vi "save_config.vi"   [LabVIEW 2011]
doc: "Illustrates how to create and write a configuration settings file.\n\nInstructions:\nEnter values in the controls on the front panel then click on the Run Arrow.\nTo read the file, run Read Configuration Settings File.vi located in the file\\config.llb."
uses:
  global.vi
  <vilib>/Utility/config.llb/Write Key (I32).vi
  <vilib>/Utility/config.llb/Write Key (Boolean).vi
  <vilib>/Utility/config.llb/Write Key (Double).vi
  <vilib>/Utility/config.llb/Write Key (String).vi
  <vilib>/Utility/config.llb/NI_LVConfig.lvlib
types:
  T1 = typedef "NI_LVConfig.lvlib/Config Data RefNum.ctl" = refnum<k1>
  T2 = typedef "scale.ctl" = dbl
  T3 = typedef "sampling_rate.ctl" = ext
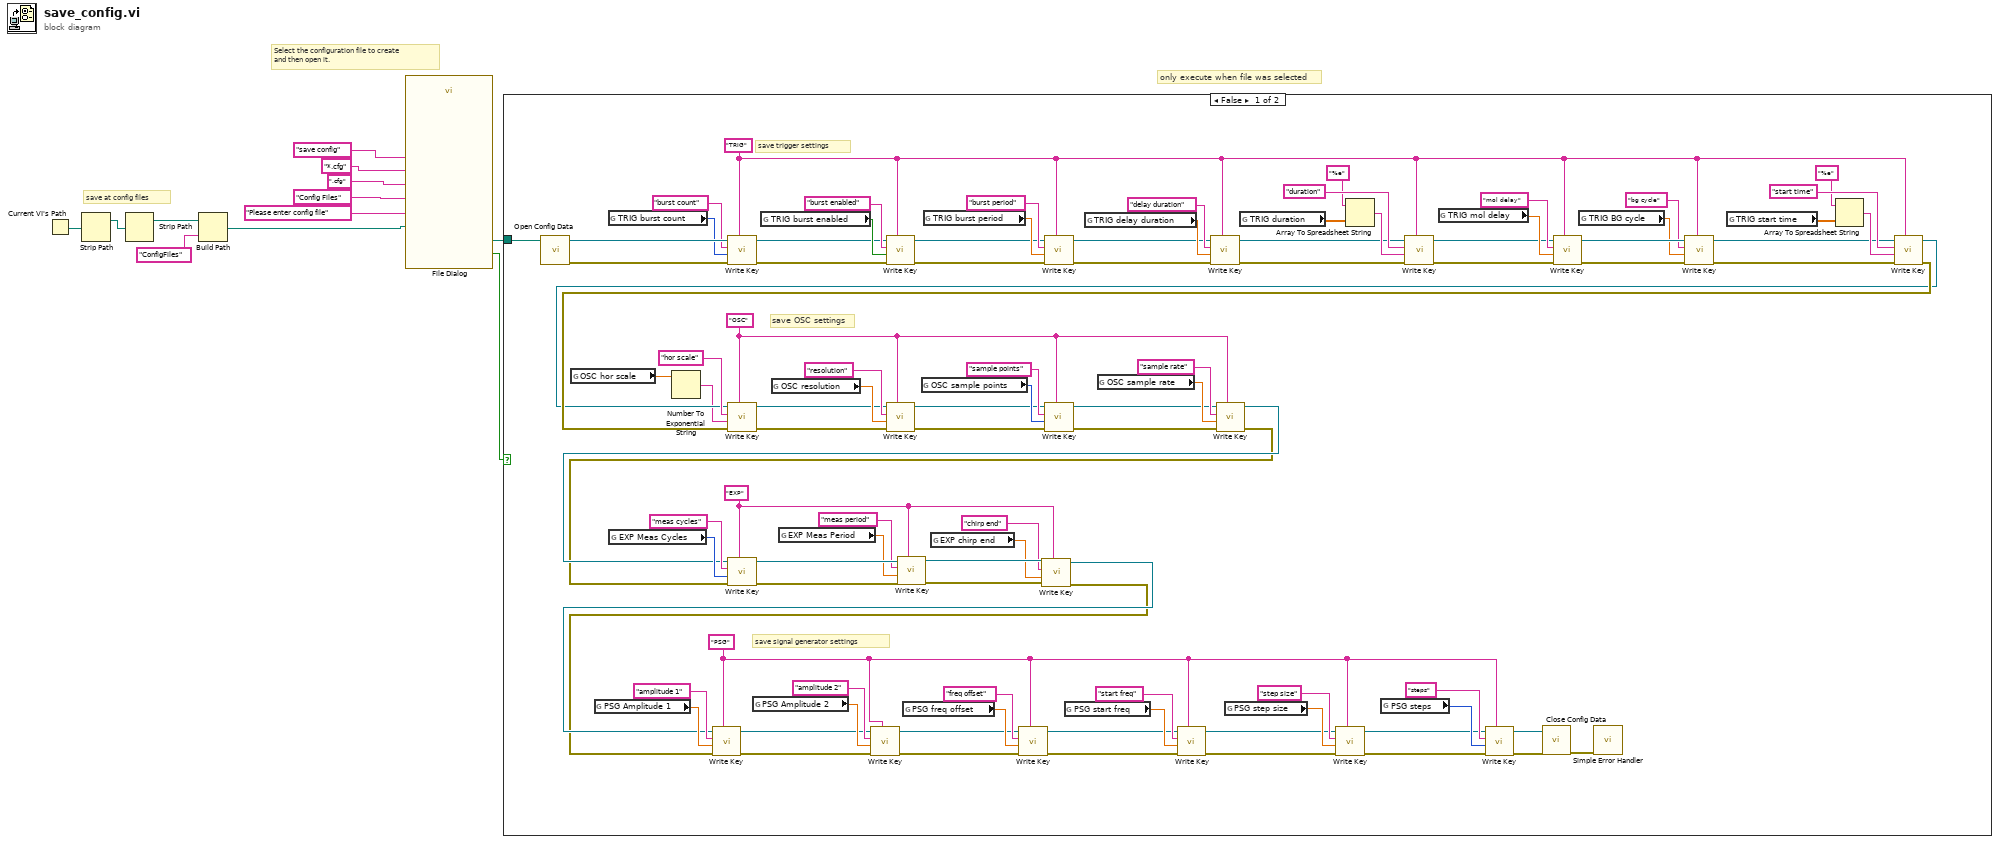
[diagram p0: block diagram]
diagram:
  # "only execute when file was selected"
  # "save at config files"
  # "Select the configuration file to create\nand then open it."
  n1 = Current VI's Path() -> (path=w6:path)
  n2 = Strip Path(path=w6) -> (stripped path=w3:path)  [unwired: 1 out]
  n3 = Strip Path(path=w3) -> (stripped path=w2:path)  [unwired: 1 out]
  n4 = Build Path(base path=w2, name or relative path="ConfigFiles") -> (appended path=w4:path)
  n5 = call "File Dialog"("start path"=w4, "prompt"="Please enter config file", "button label"="save config", "default name"=".cfg", "pattern (all files)"="*.cfg", "pattern label"="Config Files") -> ("selected path"=w12:path, "cancelled"=w1:bool)  [unwired: 6 in, 2 out]
  n6 = case shown="False" w1 {
    tunnel: w12 -> [w105 _]
    frame False {
      w32 = "PSG"
      w15 = "EXP"
      w61 = "OSC"
      w22 = "TRIG"
      # "save signal generator settings"
      # "save OSC settings"
      # "save trigger settings"
      n7 = call <vilib>:"Open Config Data.vi"("configuration file path"=w105) -> ("error out"=w108:errorcluster, "refnum"=w109:T1)  [unwired: 2 in, 7 out]
      n8 = global read "global.vi" "OSC hor scale"() -> (w31:T2)
      n9 = global read "global.vi" "PSG Amplitude 1"() -> (w42:dbl)
      n10 = global read "global.vi" "TRIG burst count"() -> (w104:i32)
      n11 = global read "global.vi" "EXP Meas Cycles"() -> (w59:i32)
      n12 = Number To Exponential String(number=w31) -> (E-format string=w30:string)  [unwired: 3 in]
      n13 = call-poly <vilib>:"Write Key.vi"("section"=w22, "error in (no error)"=w108, "value"=w104, "key"="burst count" ("Key 1"), "refnum"=w109) -> ("error out"=w89:errorcluster, "refnum out"=w93:T1)  [unwired: 5 out]
      n14 = global read "global.vi" "PSG Amplitude 2"() -> (w40:dbl)
      n15 = global read "global.vi" "TRIG burst enabled"() -> (w102:bool)
      n16 = global read "global.vi" "OSC resolution"() -> (w74:ext)
      n17 = global read "global.vi" "EXP Meas Period"() -> (w26:dbl)
      n18 = call-poly <vilib>:"Write Key.vi"("section"=w22, "error in (no error)"=w89, "value"=w102, "key"="burst enabled" ("Key 1"), "refnum"=w93) -> ("error out"=w88:errorcluster, "refnum out"=w92:T1)  [unwired: 5 out]
      n19 = global read "global.vi" "PSG freq offset"() -> (w55:dbl)
      n20 = global read "global.vi" "OSC sample points"() -> (w72:i32)
      n21 = global read "global.vi" "TRIG burst period"() -> (w100:dbl)
      n22 = global read "global.vi" "EXP chirp end"() -> (w13:dbl)
      n23 = call-poly <vilib>:"Write Key.vi"("section"=w22, "error in (no error)"=w88, "value"=w100, "key"="burst period" ("Key 1"), "refnum"=w92) -> ("error out"=w87:errorcluster, "refnum out"=w91:T1)  [unwired: 3 in, 2 out]
      n24 = global read "global.vi" "PSG start freq"() -> (w53:dbl)
      n25 = global read "global.vi" "TRIG delay duration"() -> (w98:dbl)
      n26 = global read "global.vi" "OSC sample rate"() -> (w64:T3)
      n27 = call-poly <vilib>:"Write Key.vi"("section"=w22, "error in (no error)"=w87, "value"=w98, "key"="delay duration" ("Key 1"), "refnum"=w91) -> ("error out"=w86:errorcluster, "refnum out"=w90:T1)  [unwired: 3 in, 2 out]
      n28 = global read "global.vi" "PSG step size"() -> (w51:dbl)
      n29 = global read "global.vi" "TRIG duration"() -> (w95:dbl[])
      n30 = Array To Spreadsheet String(array=w95, 3:"%e" ("format string")) -> (spreadsheet string=w94:string)  [unwired: 1 in]
      n31 = global read "global.vi" "PSG steps"() -> (w45:i32)
      n32 = call-poly <vilib>:"Write Key.vi"("section"=w22, "error in (no error)"=w86, "value"=w94, "key"="duration" ("Key 1"), "refnum"=w90) -> ("error out"=w78:errorcluster, "refnum out"=w79:T1)  [unwired: 1 in, 4 out]
      n33 = global read "global.vi" "TRIG mol delay"() -> (w80:dbl)
      n34 = call-poly <vilib>:"Write Key.vi"("section"=w22, "error in (no error)"=w78, "value"=w80, "key"="mol delay" ("Key 1"), "refnum"=w79) -> ("error out"=w77:errorcluster, "refnum out"=w24:T1)  [unwired: 3 in, 2 out]
      n35 = global read "global.vi" "TRIG BG cycle"() -> (w20:dbl)
      n36 = call-poly <vilib>:"Write Key.vi"("section"=w22, "error in (no error)"=w77, "value"=w20, "key"="bg cycle" ("Key 1"), "refnum"=w24) -> ("error out"=w25:errorcluster, "refnum out"=w23:T1)  [unwired: 4 in, 1 out]
      n37 = global read "global.vi" "TRIG start time"() -> (w83:dbl[])
      n38 = Array To Spreadsheet String(array=w83, 3:"%e" ("format string")) -> (spreadsheet string=w82:string)  [unwired: 1 in]
      n39 = call-poly <vilib>:"Write Key.vi"("section"=w22, "error in (no error)"=w25, "value"=w82, "key"="start time" ("Key 1"), "refnum"=w23) -> ("error out"=w67:errorcluster, "refnum out"=w66:T1)  [unwired: 1 in, 4 out]
      n40 = call-poly <vilib>:"Write Key.vi"("section"=w61, "error in (no error)"=w67, "value"=w30, "key"="hor scale" ("Key 1"), "refnum"=w66) -> ("error out"=w69:errorcluster, "refnum out"=w71:T1)  [unwired: 1 in, 4 out]
      n41 = call-poly <vilib>:"Write Key.vi"("section"=w61, "error in (no error)"=w69, "value"=w74, "key"="resolution" ("Key 1"), "refnum"=w71) -> ("error out"=w68:errorcluster, "refnum out"=w70:T1)  [unwired: 3 in, 2 out]
      n42 = call-poly <vilib>:"Write Key.vi"("section"=w61, "error in (no error)"=w68, "value"=w72, "key"="sample points" ("Key 1"), "refnum"=w70) -> ("error out"=w62:errorcluster, "refnum out"=w63:T1)  [unwired: 5 out]
      n43 = call-poly <vilib>:"Write Key.vi"("section"=w61, "error in (no error)"=w62, "value"=w64, "key"="sample rate" ("Key 1"), "refnum"=w63) -> ("error out"=w57:errorcluster, "refnum out"=w58:T1)  [unwired: 3 in, 2 out]
      n44 = call-poly <vilib>:"Write Key.vi"("section"=w15, "error in (no error)"=w57, "value"=w59, "key"="meas cycles" ("Key 1"), "refnum"=w58) -> ("error out"=w28:errorcluster, "refnum out"=w29:T1)  [unwired: 5 out]
      n45 = call-poly <vilib>:"Write Key.vi"("section"=w15, "error in (no error)"=w28, "value"=w26, "key"="meas period" ("Key 1"), "refnum"=w29) -> ("error out"=w18:errorcluster, "refnum out"=w19:T1)  [unwired: 3 in, 2 out]
      n46 = call-poly <vilib>:"Write Key.vi"("section"=w15, "error in (no error)"=w18, "value"=w13, "key"="chirp end" ("Key 1"), "refnum"=w19) -> ("error out"=w16:errorcluster, "refnum out"=w17:T1)  [unwired: 3 in, 2 out]
      n47 = call-poly <vilib>:"Write Key.vi"("section"=w32, "error in (no error)"=w16, "value"=w42, "key"="amplitude 1" ("Key 1"), "refnum"=w17) -> ("error out"=w38:errorcluster, "refnum out"=w39:T1)  [unwired: 3 in, 2 out]
      n48 = call-poly <vilib>:"Write Key.vi"("section"=w32, "error in (no error)"=w38, "value"=w40, "key"="amplitude 2" ("Key 1"), "refnum"=w39) -> ("error out"=w37:errorcluster, "refnum out"=w36:T1)  [unwired: 3 in, 2 out]
      n49 = call-poly <vilib>:"Write Key.vi"("section"=w32, "error in (no error)"=w37, "value"=w55, "key"="freq offset" ("Key 1"), "refnum"=w36) -> ("error out"=w48:errorcluster, "refnum out"=w50:T1)  [unwired: 3 in, 2 out]
      n50 = call-poly <vilib>:"Write Key.vi"("section"=w32, "error in (no error)"=w48, "value"=w53, "key"="start freq" ("Key 1"), "refnum"=w50) -> ("error out"=w47:errorcluster, "refnum out"=w49:T1)  [unwired: 3 in, 2 out]
      n51 = call-poly <vilib>:"Write Key.vi"("section"=w32, "error in (no error)"=w47, "value"=w51, "key"="step size" ("Key 1"), "refnum"=w49) -> ("error out"=w43:errorcluster, "refnum out"=w44:T1)  [unwired: 3 in, 2 out]
      n52 = call-poly <vilib>:"Write Key.vi"("section"=w32, "error in (no error)"=w43, "value"=w45, "key"="steps" ("Key 1"), "refnum"=w44) -> ("error out"=w34:errorcluster, "refnum out"=w35:T1)  [unwired: 5 out]
      n53 = call <vilib>:"Close Config Data.vi"("error in (no error)"=w34, "refnum"=w35) -> ("error out"=w106:errorcluster)  [unwired: 1 in, 8 out]
      n54 = call <vilib>:"Simple Error Handler.vi"("error in (no error)"=w106) -> ()  [unwired: 1 in, 8 out]
    }
    frame True {
    }
  }
